vi "onAddVerboseExplanation.vi"(5 "append":bool, 7 "overwrite":bool, 8 "error in (no error)":errorcluster, 10 "Verbose Explanation":string, 11 "Leaf.Properties in":refnum<class "Leaf.Properties.lvclass">) -> (0 "error out":errorcluster, 3 "Leaf.Properties out":refnum<class "Leaf.Properties.lvclass">)   [LabVIEW 2021, in "Banana.Caraya.lvlib" / "Leaf.Properties.lvclass"]
uses:
  Leaf.Properties.lvclass
  Leaf.Properties.lvclass/Leaf.Properties.ctl
  <vilib>/addons/_JKI Toolkits/Caraya/classes/Properties/Properties.lvclass
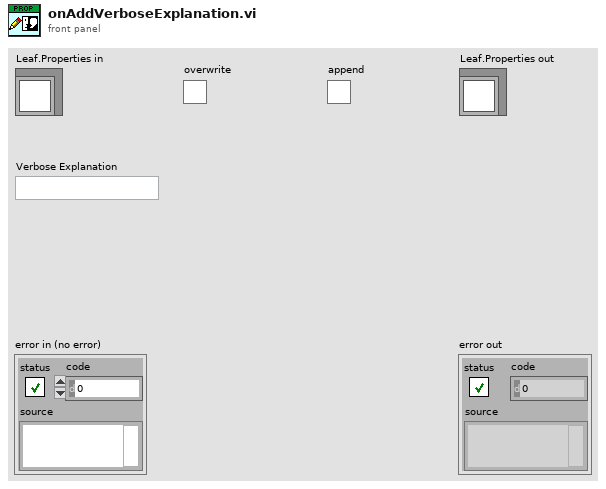
[diagram p1: front panel]
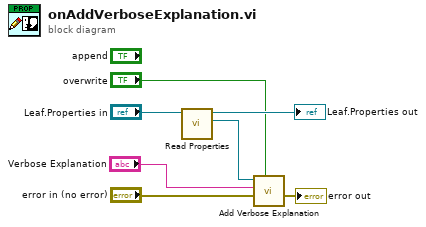
[diagram p0: block diagram]
diagram:
  n1 = call "Read Properties.vi"("Leaf.Properties in"="Leaf.Properties in") -> ("Properties"=w5:refnum<class "Properties.lvclass">, "Leaf.Properties out"=→"Leaf.Properties out":refnum<class "Leaf.Properties.lvclass">)  [unwired: 9 in]
  n2 = call <vilib>:"Add Verbose Explanation.vi"("overwrite?"="overwrite", "error in (no error)"="error in (no error)", "Verbose Explanation"="Verbose Explanation", "Properties"=w5) -> ("error out"=→"error out":errorcluster)  [unwired: 6 in, 1 out]
